vi "forebrainRequestForMidbrain.vi"(1 "Rudder Angle":i16) -> (0 "output array":dbl[](array[numeric]))   [LabVIEW 2012]
panel:
  out "Rudder Angle Desire":dbl[](graph)
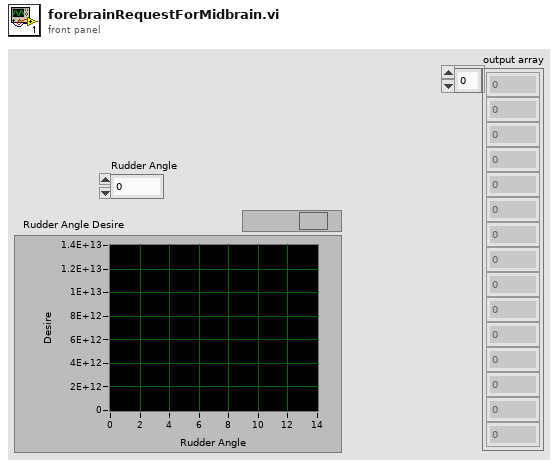
[diagram p1: front panel]
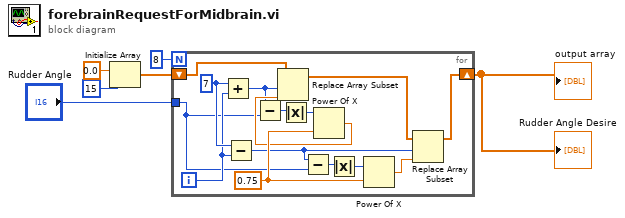
[diagram p0: block diagram]
diagram:
  n1 = Initialize Array(0.0 ("element"), 15 ("dimension size")) -> (w2:dbl[])
  n2 = for {
    N: 8 -> [_]
    tunnel: "Rudder Angle" -> [w9]
    shift-right: [w17] -> w1
    shift-left: w2 -> [w19]
    i -> [w20]
    w16 = 0.75 ("x")
    w21 = 7
    n3 = Add(x=w21, y=w20) -> (x+y=w8:i32)
    n4 = Subtract(x=w21, y=w20) -> (x-y=w7:i32)
    n5 = Subtract(x=w8, y=w9) -> (x-y=w15:i32)
    n6 = Absolute Value(x=w15) -> (abs(x)=w14:i32)
    n7 = Subtract(x=w7, y=w9) -> (x-y=w11:i32)
    n8 = Power Of X(1:w16, 2:w14) -> (0:w13:dbl)
    n9 = Replace Array Subset(array=w19, new element=w13, index=w8) -> (w18:dbl[])
    n10 = Absolute Value(x=w11) -> (abs(x)=w10:i32)
    n11 = Power Of X(1:w16, 2:w10) -> (0:w12:dbl)
    n12 = Replace Array Subset(array=w18, new element=w12, index=w7) -> (w17:dbl[])
  }
  "output array" <- w1
  "Rudder Angle Desire" <- w1
